vi "DB_DataChg.vi"(8 "错误输入（无错误）":errorcluster, 11 "data":variant[][](array[variant])) -> (0 "错误输出":errorcluster, 3 "数组":string[][](array[string]))   [LabVIEW 2016]
uses:
  Insertdata.ctl
  <vilib>/addons/database/_DB Variant To Data/Database Variant To Data.xnode
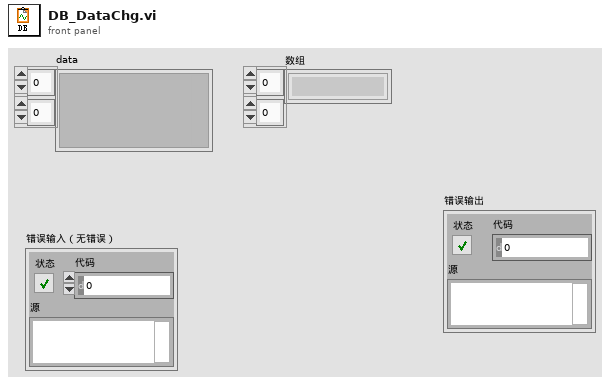
[diagram p1: front panel]
types:
  T1 = typedef "Insertdata.ctl" = cluster{"Identity":i32, "Time":string, "Meaning":string, "Thumb":i32, "Index":i32, "Middle":i32, "ring":i32, "little":i32, "wrist":i32, "arm":i32, "rota":i32, "delay":i32}
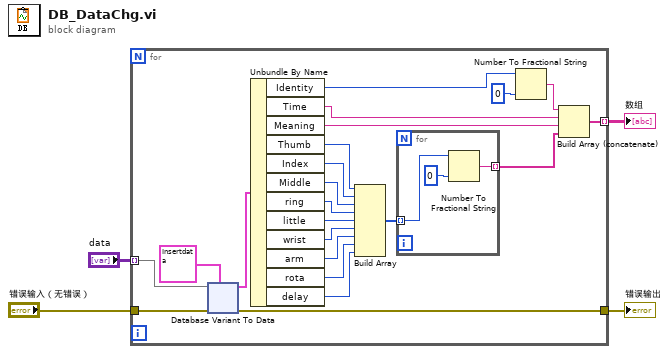
[diagram p0: block diagram]
diagram:
  n1 = for {
    tunnel: "data" -> [w26] mode=indexing
    tunnel: [w25] -> w2 mode=indexing
    tunnel: "错误输入（无错误）" -> [w22]
    tunnel: [w21] -> w4
    n2 = xnode "Database Variant To Data"("database variant"=w26, "error in (no error)"=w22, "type"=T1 {"Identity"=1, "Time"="俞忠达", "Meaning"="语义", "Thumb"=1, "Index"=1, "Middle"=1, "ring"=1, "little"=1, "wrist"=1, "arm"=1, "rota"=1, "delay"=1} ("Data")) -> ("data"=w19:T1, "error out"=w21:errorcluster)
    n3 = Unbundle By Name(w19) -> ("Identity"=w18:i32, "Time"=w17:string, "Meaning"=w16:string, "Thumb"=w12:i32, "Index"=w13:i32, "Middle"=w14:i32, "ring"=w15:i32, "little"=w11:i32, "wrist"=w10:i32, "arm"=w9:i32, "rota"=w8:i32, "delay"=w7:i32)
    n4 = Build Array(w12, w13, w14, w15, w11, w10, w9, w8, w7) -> (w6:i32[])
    n5 = for {
      tunnel: w6 -> [w28] mode=indexing
      tunnel: [w27] -> w5 mode=indexing
      n6 = Number To Fractional String(number=w28, precision (6)=i16 0 ("精度(6)")) -> (F-format string=w27:string)  [unwired: 2 in]
    }
    n7 = Number To Fractional String(number=w18, precision (6)=i16 0 ("精度(6)")) -> (F-format string=w24:string)  [unwired: 2 in]
    n8 = Build Array (concatenate)(w24, w17, w16, w5) -> (w25:string[])
  }
  "错误输出" <- w4
  "数组" <- w2
